vi "test_Check String Comparison_error in goes through.vi"(8 "error in (no error)":errorcluster, 11 "TestCase in":refnum<class "Instrument Addon Unit Tests.lvclass">) -> (0 "error out":errorcluster, 3 "TestCase out":refnum<class "Instrument Addon Unit Tests.lvclass">)   [LabVIEW 2018, in "Instrument Addon Unit Tests.lvclass"]
uses:
  Instrument Addon Unit Tests.lvclass
  <vilib>/addons/_JKI Toolkits/VI Tester/TestCase.llb/TestCase.lvclass
  Addon/Addon Engine/Instrument Addon Engine.lvlib
  C:/Program Files (x86)/National Instruments/LabVIEW 2018/vi.lib/addons/_JKI Toolkits/VI Tester/TestCase.llb/TestCase.lvclass
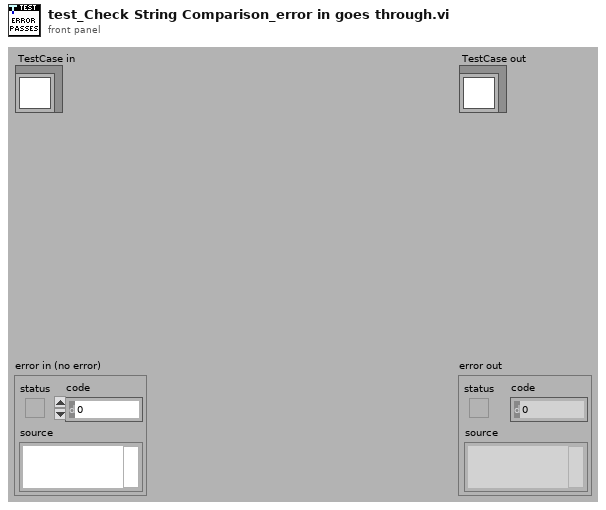
[diagram p1: front panel]
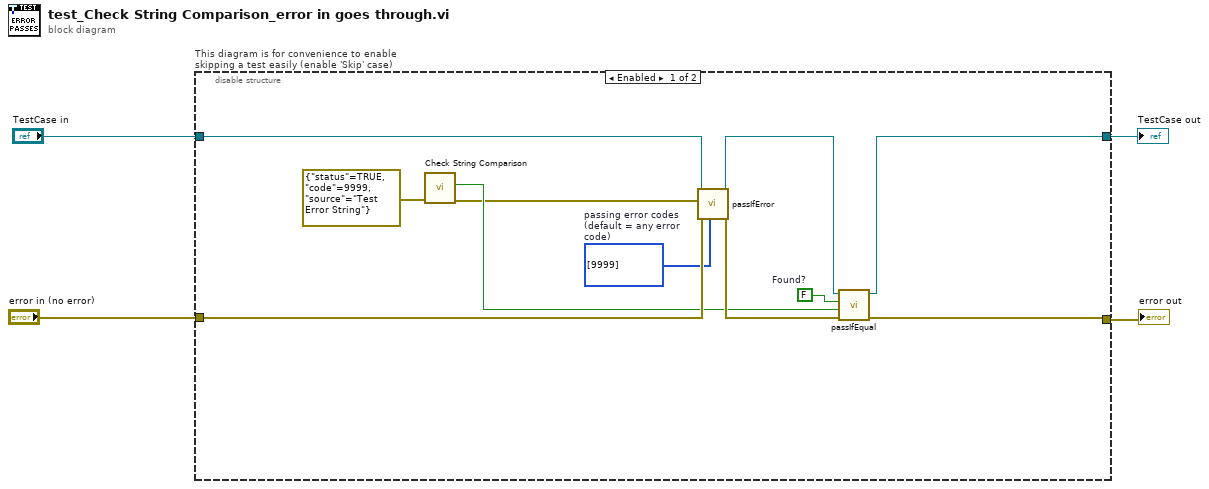
[diagram p0: block diagram]
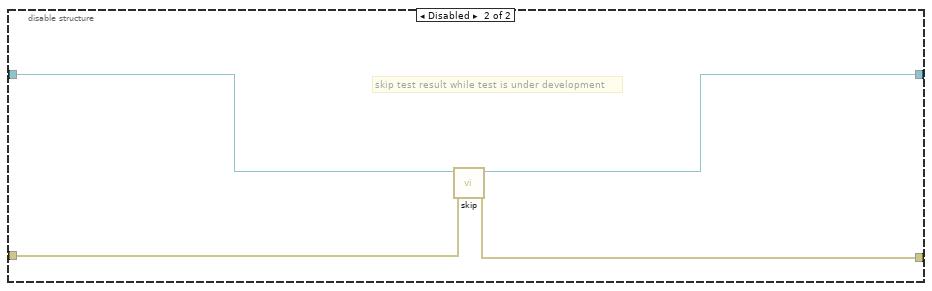
[diagram p2: hidden frame]
diagram:
  n1 = disable-structure "This diagram is for convenience to enable skipping a test easily (enable 'Skip' case)" shown="Enabled" {
    disable-tunnel: "TestCase in" -> [w15 w19]
    disable-tunnel: [w10 w17] -> w1
    disable-tunnel: [w13 w18] -> w3
    disable-tunnel: "error in (no error)" -> [w9 w16]
    frame Enabled {
      w5 = i32[] [9999]  # passing error codes (default = any error code)
      w12 = FALSE  # Found?
      n2 = call "Check String Comparison.vi"("error in (no error)"=errorcluster {"status"=TRUE, "code"=9999, "source"="Test Error String"}) -> ("error out"=w6:errorcluster, "Found?"=w7:bool)  [unwired: 8 in, 1 out]
      n3 = call-dynamic "passIfError.vi"("passing error codes (default = any error code)"=w5, "error in (no error)"=w9, "error"=w6, "TestCase in"=w15) -> ("error out"=w14:errorcluster, "TestCase out"=w11:refnum<class "Instrument Addon Unit Tests.lvclass">)  [unwired: 6 in]
      n4 = call-dynamic "passIfEqual.vi"("error in (no error)"=w14, "y"=w7, "x"=w12, "TestCase in"=w11) -> ("error out"=w13:errorcluster, "TestCase out"=w10:refnum<class "Instrument Addon Unit Tests.lvclass">)  [unwired: 6 in]
    }
    frame Disabled {
      # "skip test result while test is under development"
      n5 = call <vilib>:"skip.vi"("error in (no error)"=w16, "TestCase in"=w19) -> ("error out"=w18:errorcluster, "TestCase out"=w17:refnum<class "Instrument Addon Unit Tests.lvclass">)  [unwired: 8 in]
    }
  }
  "error out" <- w3
  "TestCase out" <- w1
